vi "[Example] List Package Attributes in NIPB Solution.vi"() -> ()   [LabVIEW 2017]
uses:
  NIPB Solution API/NIPB Solution API.lvlib
panel:
  out "Package Names":string[](array[string])
  out "Package Categories":string[](array[string])
  out "Package Versions":string[](array[string])
  in  "NI Package Builder solution (.pbs)":path
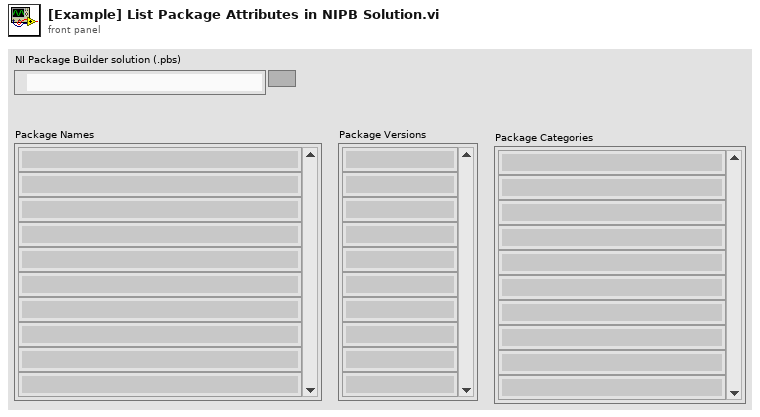
[diagram p1: front panel]
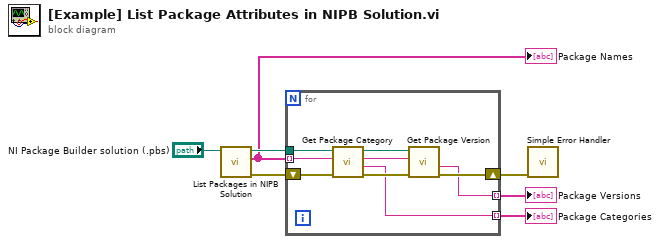
[diagram p0: block diagram]
diagram:
  n1 = call "List Packages in NIPB Solution.vi"("NI Package Builder solution (.pbs)"="NI Package Builder solution (.pbs)") -> ("error out"=w5:errorcluster, "package names"=w4:string[], "NI Package Builder solution out"=w6:path)  [unwired: 8 in]
  "Package Names" <- w4
  n2 = for {
    tunnel: w6 -> [w16]
    shift-right: [w12] -> w1
    shift-left: w5 -> [w15]
    tunnel: w4 -> [w13] mode=indexing
    tunnel: [w9] -> w3 mode=indexing
    tunnel: [w8] -> w2 mode=indexing
    n3 = call "Get Package Category.vi"("error in (no error)"=w15, "package name"=w13, "NI Package Builder solution (.pbs)"=w16) -> ("error out"=w14:errorcluster, "category"=w8:string, "package name out"=w10:string, "NI Package Builder solution out"=w11:path)  [unwired: 5 in]
    n4 = call "Get Package Version.vi"("error in (no error)"=w14, "package name"=w10, "NI Package Builder solution (.pbs)"=w11) -> ("error out"=w12:errorcluster, "version"=w9:string)  [unwired: 5 in, 2 out]
  }
  "Package Versions" <- w3
  "Package Categories" <- w2
  n5 = call <vilib>:"Simple Error Handler.vi"("error in (no error)"=w1) -> ()  [unwired: 4 in, 5 out]
